vi "Character Data To Images.vi"(1 "All Rows of Data":dbl[][](array[numeric])) -> (0 "Character Images":picture[](array[picture]))   [LabVIEW 2015]
uses:
  <vilib>/picture/picture.llb/Draw True-Color Pixmap.vi
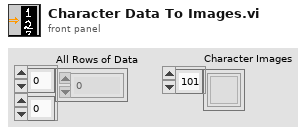
[diagram p1: front panel]
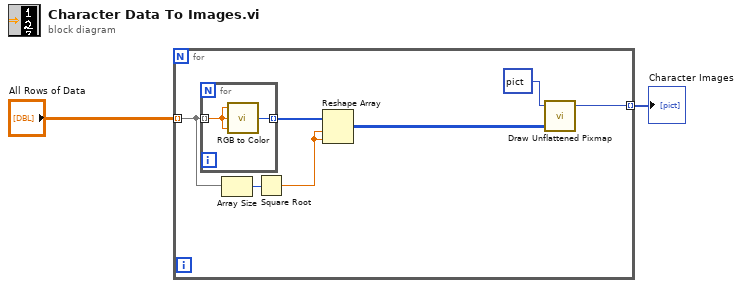
[diagram p0: block diagram]
diagram:
  n1 = for {
    tunnel: "All Rows of Data" -> [w5] mode=indexing
    tunnel: [w6] -> w2 mode=indexing
    n2 = for {
      tunnel: w5 -> [w11] mode=indexing
      tunnel: [w10] -> w9 mode=indexing
      n3 = call <vilib>:"RGB to Color.vi"("B"=w11, "G"=w11, "R"=w11) -> ("Color"=w10:u32)
    }
    n4 = Array Size(array=w5) -> (size(s)=w4:i32)
    n5 = Square Root(x=w4) -> (sqrt(x)=w3:dbl)
    n6 = Reshape Array(w9, w3, w3) -> (w8:u32[][])
    n7 = call-poly <vilib>:"Draw Unflattened Pixmap.vi"("picture"=picture data[5B], "data (RGB format)"=w8) -> ("new picture"=w6:picture)  [unwired: 7 in]
  }
  "Character Images" <- w2
